vi "Laser power controller (No Objects).vi"(8 "error in (no error)":errorcluster, 11 "VISA Resource Name":refnum<visa-resource-name>="GPIB0::3::INSTR") -> (0 "error out":errorcluster, 3 "Cluster out":T1)   [LabVIEW 2009]
panel:
  out "Status":string
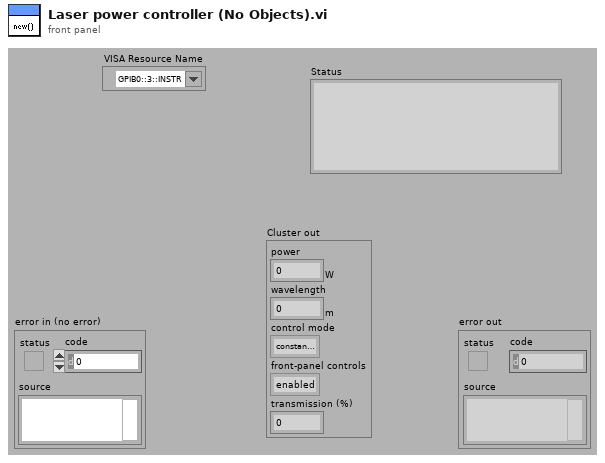
[diagram p1: front panel]
types:
  T1 = cluster{"power":dbl[unit], "wavelength":dbl[unit], "control mode":enum16{"constant power", "constant transmission"}, "front-panel controls":enum16{"enabled", "disabled"}, "transmission (%)":dbl}
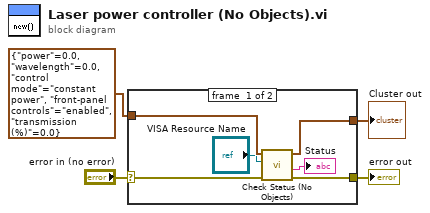
[diagram p0: block diagram]
diagram:
  n1 = case shown="No Error" "error in (no error)" {
    selector: "error in (no error)" -> [w7 w12]
    tunnel: [w9 w12] -> w3
    tunnel: [w10 w11] -> w1
    tunnel: T1 {"power"=0.0, "wavelength"=0.0, "control mode"=enum."constant power", "front-panel controls"=enum."enabled", "transmission (%)"=0.0} ("Cluster of class private data") -> [w6 w11]
    frame #0 {
      n2 = call "Check Status (No Objects).vi"("error in (no error)"=w7, "VISA Resource Name"="VISA Resource Name", "Cluster In"=w6) -> ("error out"=w9:errorcluster, "Status"=→"Status":string, "Cluster Out"=w10:T1)  [unwired: 5 in, 1 out]
    }
    frame #1 {
    }
  }
  "error out" <- w3
  "Cluster out" <- w1
